vi "GaussianFit2D.vi"(5 "Image":dbl[][](graph)) -> (0 "b":dbl format="%.2f", 1 "y":dbl format="%.2f", 2 "theta":dbl[unit] format="%.2f", 3 "a":dbl format="%.2f", 4 "x":dbl format="%.2f")   [LabVIEW 2009]
panel:
  # "Parameters a and b are defined as:\ne^(-x^2/a^2-y^2/b^2)"
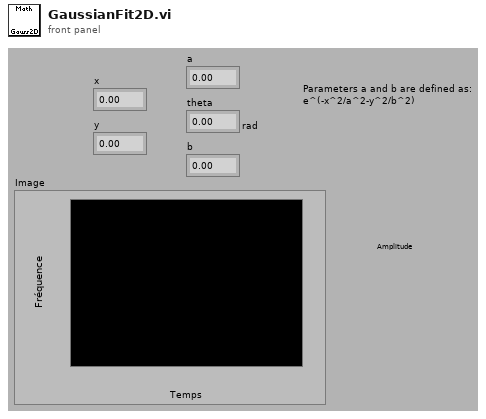
[diagram p1: front panel]
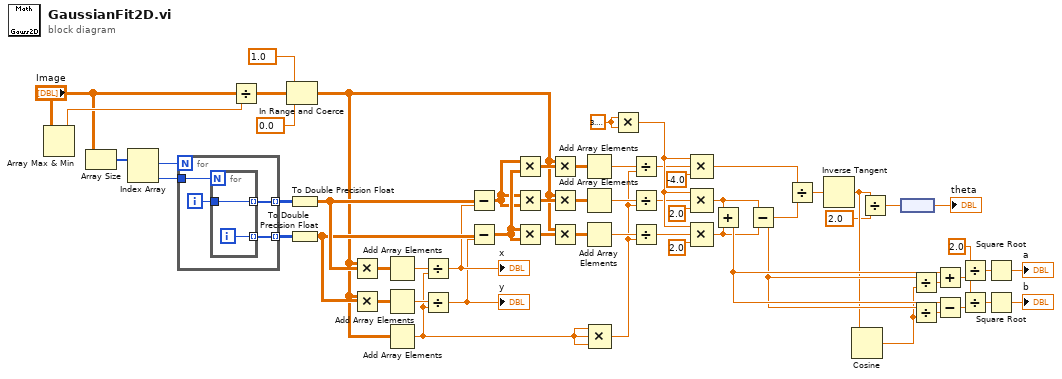
[diagram p0: block diagram]
diagram:
  w33 = 3.141592653589793
  w59 = 2.0 ("y")
  n1 = Array Max & Min(array="Image") -> (max value=w7:dbl)  [unwired: 3 out]
  n2 = Array Size(array="Image") -> (size(s)=w29:i32[])
  n3 = Index Array(array=w29) -> (element #1=w30:i32, element #2=w31:i32)  [unwired: 2 in]
  n4 = for {
    N: w30 -> [_]
    tunnel: w31 -> [w64]
    tunnel: [w63] -> w11 mode=indexing
    tunnel: [w61] -> w12 mode=indexing
    i -> [w62]
    n5 = for {
      N: w64 -> [_]
      tunnel: [w66] -> w63 mode=indexing
      tunnel: w62 -> [w66]
      tunnel: [w65] -> w61 mode=indexing
      i -> [w65]
    }
  }
  n6 = Divide(x="Image", y=w7) -> (x/y=w8:dbl[][])
  n7 = In Range and Coerce(upper limit=1.0, x=w8, lower limit=0.0) -> (coerced(x)=w6:dbl[][])  [unwired: 1 out]
  n8 = To Double Precision Float(number=w11) -> (double precision float=w18:dbl[][])
  n9 = To Double Precision Float(number=w12) -> (double precision float=w13:dbl[][])
  n10 = Multiply(x=w6, y=w18) -> (x*y=w14:dbl[][])
  n11 = Multiply(x=w6, y=w13) -> (x*y=w15:dbl[][])
  n12 = Add Array Elements(numeric array=w14) -> (sum=w17:dbl)
  n13 = Add Array Elements(numeric array=w15) -> (sum=w16:dbl)
  n14 = Add Array Elements(numeric array=w6) -> (sum=w9:dbl)
  n15 = Divide(x=w17, y=w9) -> (x/y=w2:dbl)
  "x" <- w2
  n16 = Divide(x=w16, y=w9) -> (x/y=w1:dbl)
  "y" <- w1
  n17 = Subtract(x=w18, y=w2) -> (x-y=w23:dbl[][])
  n18 = Subtract(x=w13, y=w1) -> (x-y=w24:dbl[][])
  n19 = Multiply(x=w23, y=w24) -> (x*y=w25:dbl[][])
  n20 = Multiply(x=w23, y=w23) -> (x*y=w19:dbl[][])
  n21 = Multiply(x=w24, y=w24) -> (x*y=w20:dbl[][])
  n22 = Multiply(x=w6, y=w25) -> (x*y=w26:dbl[][])
  n23 = Multiply(x=w6, y=w19) -> (x*y=w21:dbl[][])
  n24 = Multiply(x=w6, y=w20) -> (x*y=w22:dbl[][])
  n25 = Add Array Elements(numeric array=w26) -> (sum=w28:dbl)
  n26 = Add Array Elements(numeric array=w21) -> (sum=w27:dbl)
  n27 = Add Array Elements(numeric array=w22) -> (sum=w32:dbl)
  n28 = Compound Arithmetic op=MULTIPLY(w9, w9, w9) -> (w10:dbl)
  n29 = Multiply(x=w33, y=w33) -> (x*y=w37:dbl)
  n30 = Divide(x=w28, y=w10) -> (x/y=w34:dbl)
  n31 = Divide(x=w27, y=w10) -> (x/y=w35:dbl)
  n32 = Divide(x=w32, y=w10) -> (x/y=w36:dbl)
  n33 = Compound Arithmetic op=MULTIPLY(w37, w34, -4.0) -> (w41:dbl)
  n34 = Compound Arithmetic op=MULTIPLY(w37, w35, 2.0) -> (w42:dbl)
  n35 = Compound Arithmetic op=MULTIPLY(w37, w36, 2.0) -> (w43:dbl)
  n36 = Add(x=w42, y=w43) -> (x+y=w56:dbl)
  n37 = Subtract(x=w42, y=w43) -> (x-y=w55:dbl)
  n38 = Divide(x=w41, y=w55) -> (x/y=w44:dbl)
  n39 = Inverse Tangent(1:w44) -> (0:w48:dbl)
  n40 = Cosine(x=w48) -> (cos(x)=w54:dbl)
  n41 = Divide(x=w48, y=2.0) -> (x/y=w46:dbl)
  n42 = node(w46) -> (→"theta":dbl[unit])
  n43 = Divide(x=w55, y=w54) -> (x/y=w53:dbl)
  n44 = Divide(x=w55, y=w54) -> (x/y=w52:dbl)
  n45 = Add(x=w56, y=w53) -> (x+y=w49:dbl)
  n46 = Subtract(x=w56, y=w52) -> (x-y=w58:dbl)
  n47 = Divide(x=w59, y=w49) -> (x/y=w50:dbl)
  n48 = Divide(x=w59, y=w58) -> (x/y=w57:dbl)
  n49 = Square Root(x=w50) -> (sqrt(x)=→"a":dbl)
  n50 = Square Root(x=w57) -> (sqrt(x)=→"b":dbl)
